vi "SSC Relay Expand Action Array to All Sessions.vi"(0 "SSC Relay in":T2[](array[typedef]), 7 "Relay Actions in":T1[](array[typedef]) items=["Open Relay"=20, "Close Relay"=21], 11 "error in":errorcluster) -> (4 "SSC Relay out":T2[](array[typedef]), 8 "Relay Actions out":T1[](array[typedef]) items=["Open Relay"=20, "Close Relay"=21], 15 "error out":errorcluster)   [LabVIEW 2019]
doc: "This VI expands the Relay Actions array to provide one action per SSC session.\n\nCases:\n-If the array is empty this function generates an array of default type and throws an error\n-If the array has one element the function maps it to all sessions\n-If the array is an even multiple size of the number of sessions it maps the array multiple times (used to expand across sites)\n-If the array is not an even multiple size the function maps the array and throws a warning\n-If the array is the same size as the sessions it passes it straight through\n-If the aray is larger than the sessions it gets shortened and a warning is emitted"
uses:
  SSC Relay.ctl
  <instrlib>/niSwitch/niSwitch.llb/niSwitch Relay Action.ctl
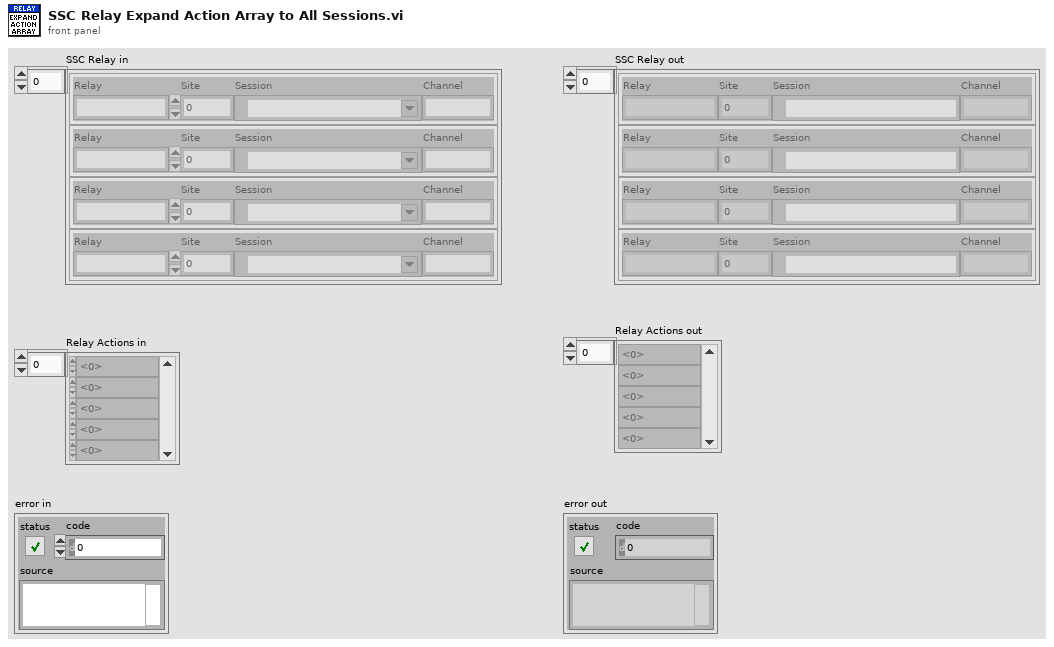
[diagram p1: front panel]
types:
  T1 = typedef "niSwitch Relay Action.ctl" = i32
  T2 = typedef "SSC Relay.ctl" = cluster{"Relay":string, "Site":i32, "Session":refnum<k15>, "Channel":string}
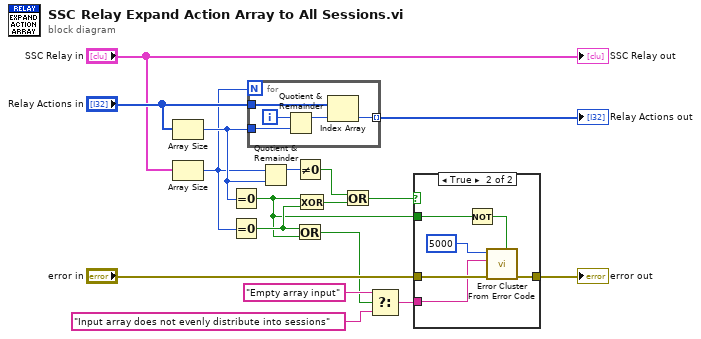
[diagram p0: block diagram]
diagram:
  n1 = Array Size(array="Relay Actions in") -> (size(s)=w9:i32)
  n2 = Array Size(array="SSC Relay in") -> (size(s)=w3:i32)
  n3 = Equal To 0?(x=w9) -> (x = 0?=w4:bool)
  n4 = Equal To 0?(x=w3) -> (x = 0?=w7:bool)
  n5 = for {
    N: w3 -> [_]
    tunnel: "Relay Actions in" -> [w22]
    tunnel: w9 -> [w20]
    tunnel: [w19] -> w2 mode=indexing
    i -> [w21]
    n6 = Quotient & Remainder(x=w21, y=w20) -> (x-y*floor(x/y)=w18:i32)  [unwired: 1 out]
    n7 = Index Array(array=w22, index=w18) -> (element=w19:T1)
  }
  "Relay Actions out" <- w2
  n8 = Quotient & Remainder(x=w3, y=w9) -> (x-y*floor(x/y)=w14:i32)  [unwired: 1 out]
  n9 = Not Equal To 0?(x=w14) -> (x != 0?=w10:bool)
  n10 = Or(x=w7, y=w4) -> (x .or. y?=w8:bool)
  n11 = Exclusive Or(1:w7, 2:w4) -> (0:w6:bool)
  n12 = Or(x=w10, y=w6) -> (x .or. y?=w15:bool)
  n13 = Select(t="Empty array input", s=w8, f="Input array does not evenly distribute into sessions") -> (s? t:f=w13:string)
  n14 = case shown="True" w15 {
    tunnel: "error in" -> [w23 w29]
    tunnel: [w23 w28] -> w16
    tunnel: w13 -> [_ w26]
    tunnel: w4 -> [_ w25]
    frame False {
    }
    frame True {
      n15 = Not(x=w25) -> (.not. x?=w24:bool)
      n16 = call <vilib>:"Error Cluster From Error Code.vi"("is warning? (False)"=w24, "error in (no error)"=w29, "error message (\"\")"=w26, "error code (0)"=5000) -> ("error out"=w28:errorcluster)  [unwired: 5 in]
    }
  }
  "error out" <- w16
  "SSC Relay out" <- "SSC Relay in"
